vi "Wait On Occurrence.vi"(8 "error in":errorcluster, 11 "occurrence in":refnum<k4>) -> (0 "error out":errorcluster)   [LabVIEW 2019, in "grpc-lvsupport.lvlib"]
uses:
  grpc-lvsupport.lvlib
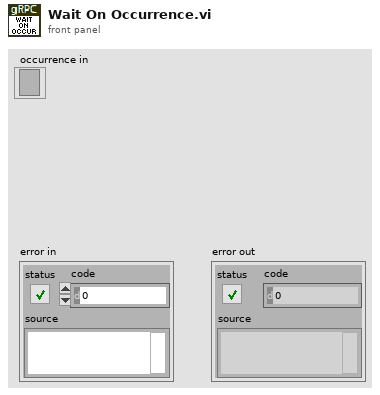
[diagram p1: front panel]
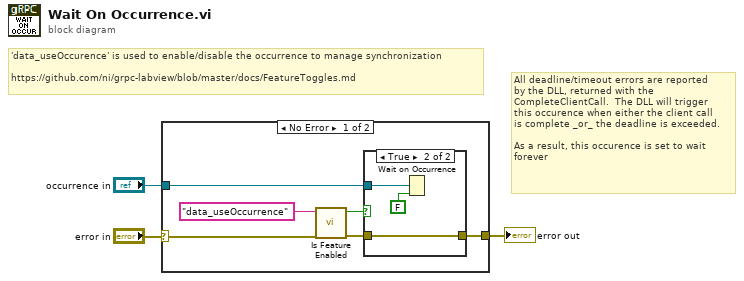
[diagram p0: block diagram]
diagram:
  # "All deadline/timeout errors are reported\nby the DLL, returned with the \nCompleteClientCall.  The DLL will trigger\nthis occurence when either the client call\nis complete _or_ the deadline is exceeded.\n\nAs a result, this occurence is set to wait\nforever"
  # "'data_useOccurence' is used to enable/disable the occurrence to manage synchronization\n\nhttps://github.com/ni/grpc-labview/blob/master/docs/FeatureToggles.md"
  n1 = case shown="No Error" "error in" {
    selector: "error in" -> [w7 w14]
    tunnel: [w5 w14] -> w2
    tunnel: "occurrence in" -> [w9 _]
    frame No Error {
      n2 = call "Is Feature Enabled.vi"("error in"=w7, "feature name"="data_useOccurrence" ("key")) -> ("error out"=w6:errorcluster, "feature enabled?"=w4:bool)  [unwired: 8 in]
      n3 = case shown="True" w4 {
        tunnel: w9 -> [_ w13]
        tunnel: [w10 w11] -> w5
        tunnel: w6 -> [w10 w11]
        frame False {
        }
        frame True {
          n4 = Wait on Occurrence(1:FALSE ("ignore previous (T)"), 2:w13) -> ()  [unwired: 1 in, 1 out]
        }
      }
    }
    frame Error {
    }
  }
  "error out" <- w2
